vi "PDC_GetTransferOption.vi"(0 "DeviceNo":u32, 5 "ChildNo":u32, 11 "error in (no error)":errorcluster) -> (4 "ReturnValue":u32, 6 "8BitSel":u32, 8 "Bayer":u32, 10 "Interleave":u32, 14 "ErrorCode":u32, 15 "error out":errorcluster)   [LabVIEW 2015]
doc: "This VI retrieves the setting condition of the image data transfer option."
uses:
  PDCLIB.dll
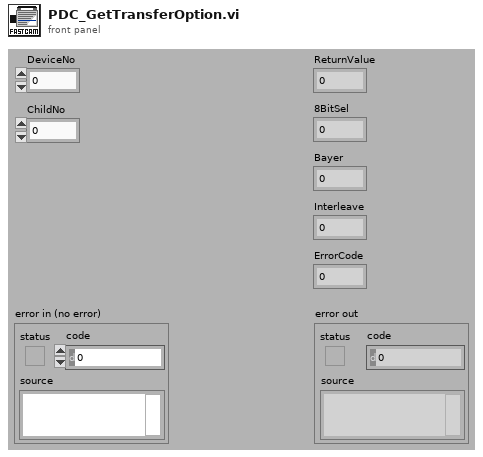
[diagram p1: front panel]
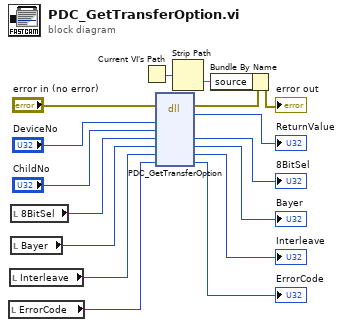
[diagram p0: block diagram]
diagram:
  n1 = local read "ErrorCode"() -> (w13:u32)
  n2 = local read "Interleave"() -> (w7:u32)
  n3 = local read "8BitSel"() -> (w9:u32)
  n4 = local read "Bayer"() -> (w8:u32)
  n5 = Current VI's Path() -> (path=w3:path)
  n6 = dll-call lib="PDCLIB.dll" fn="PDC_GetTransferOption"(error in="error in (no error)", "nDeviceNo"="DeviceNo", "nChildNo"="ChildNo", "p8BitSel"=w9, "pBayer"=w8, "pInterleave"=w7, "pErrorCode"=w13) -> (error out=w2:errorcluster, "return type"=→"ReturnValue":u32, "p8BitSel"=→"8BitSel":u32, "pBayer"=→"Bayer":u32, "pInterleave"=→"Interleave":u32, "pErrorCode"=→"ErrorCode":u32)  [unwired: 4 in, 1 out]
  n7 = Strip Path(path=w3) -> (name=w4:string)  [unwired: 1 out]
  n8 = Bundle By Name(cluster=w2, "source"=w4) -> (→"error out":errorcluster)
